vi "tempconvert.vi"() -> ()   [LabVIEW 2020]
uses:
  tempenum.ctl
panel:
  out "Ühik":string
  out "Temp":dbl
  in  "Mis ühikusse?":T1=enum."Fahrenheit"
  in  "Temp (K)":dbl
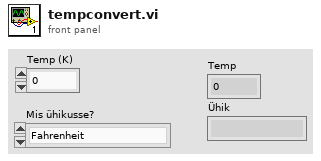
[diagram p1: front panel]
types:
  T1 = typedef "tempenum.ctl" = enum16{"Kelvin", "Fahrenheit", "Celsius"}
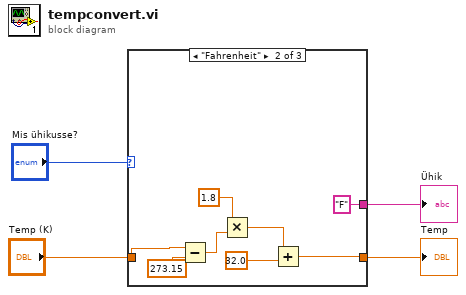
[diagram p0: block diagram]
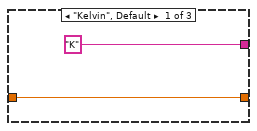
[diagram p2: hidden frame]
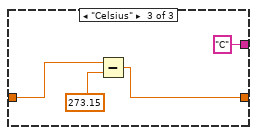
[diagram p3: hidden frame]
diagram:
  n1 = case shown="\"Fahrenheit\"" "Mis ühikusse?" {
    tunnel: "Temp (K)" -> [w6 w13 w17]
    tunnel: [w6 w7 w16] -> w2
    tunnel: ["K" "F" "C"] -> w1
    frame "Kelvin", Default {
    }
    frame "Fahrenheit" {
      n2 = Subtract(x=w13, y=273.15) -> (x-y=w11:dbl)
      n3 = Multiply(x=1.8, y=w11) -> (x*y=w9:dbl)
      n4 = Add(x=w9, y=32.0) -> (x+y=w7:dbl)
    }
    frame "Celsius" {
      n5 = Subtract(x=w17, y=273.15 ("x")) -> (x-y=w16:dbl)
    }
  }
  "Temp" <- w2
  "Ühik" <- w1
